vi "Do.vi"(8 "error in (no error)":errorcluster, 10 "Actor in":refnum<class "Actor.lvclass">, 11 "Update Status Log Msg":refnum<class "Update Status Log Msg.lvclass">) -> (0 "error out":errorcluster, 2 "Actor out":refnum<class "Actor.lvclass">)   [LabVIEW 2019, in "Chat Window Model.lvlib" / "Update Status Log Msg.lvclass"]
doc: "This VI delivers the message to the actor by calling the appropriate method(s) on the actor."
uses:
  Update Status Log Msg.lvclass
  <vilib>/ActorFramework/Actor/Actor.lvclass
  Chat Window Model/Chat Window Model.lvclass
  C:/Program Files/National Instruments/LabVIEW 2019/vi.lib/ActorFramework/Actor/Actor.lvclass
  Update Status Log Msg.lvclass/Update Status Log Msg.ctl
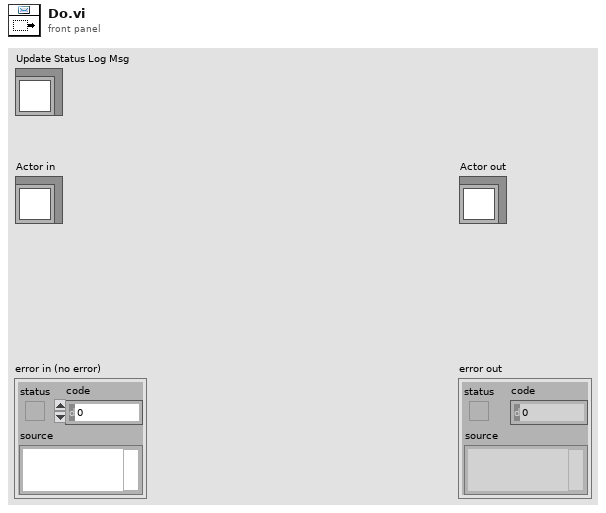
[diagram p1: front panel]
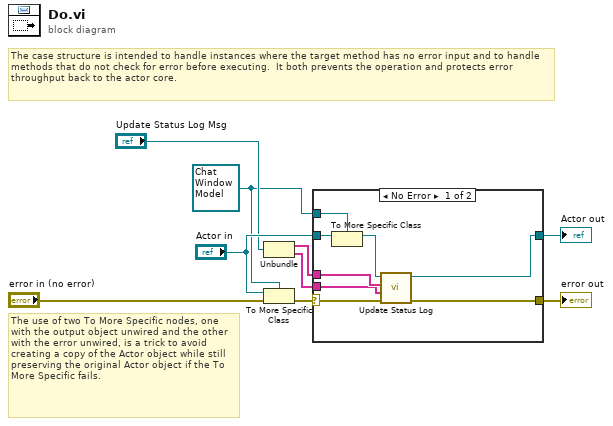
[diagram p0: block diagram]
diagram:
  w4 = refnum<class "Chat Window Model.lvclass"> refnum ("Actor in")
  # "The use of two To More Specific nodes, one with the output object unwired and the other with the error unwired, is a trick to avoid creating a copy of the Actor object while still preserving the original Actor object if the To More Specific fails."
  # "The case structure is intended to handle instances where the target method has no error input and to handle methods that do not check for error before executing.  It both prevents the operation and protects error throughput back to the actor core."
  n1 = Unbundle("Update Status Log Msg") -> (w2:string[], w1:string[])
  n2 = To More Specific Class(target class=w4, reference="Actor in", error in="error in (no error)") -> (error out=w3:errorcluster)  [unwired: 1 out]
  n3 = case shown="No Error" w3 {
    selector: w3 -> [w15 w19]
    tunnel: [w17 w19] -> w9
    tunnel: [w16 w18] -> w8
    tunnel: "Actor in" -> [w14 w18]
    tunnel: w4 -> [w13 _]
    tunnel: w2 -> [w11 _]
    tunnel: w1 -> [w10 _]
    frame No Error {
      n4 = To More Specific Class(target class=w13, reference=w14) -> (specific class reference=w12:refnum<class "Chat Window Model.lvclass">)  [unwired: 1 in, 1 out]
      n5 = call "Update Status Log.vi"("error in (no error)"=w15, "Status List"=w10, "Names"=w11, "Chat Window Model in"=w12) -> ("error out"=w17:errorcluster, "Chat Window Model out"=w16:refnum<class "Chat Window Model.lvclass">)  [unwired: 6 in]
    }
    frame Error {
      # "If type check fails, pass the original object out again."
    }
  }
  "error out" <- w9
  "Actor out" <- w8
